vi "Sort-To-XYZ-PRO.vi"(9 "位置 2":i32, 11 "位置":i32) -> (1 "移動二":dbl[](array[numeric]), 3 "移動一":dbl[](array[numeric]), 5 "放球校正?":bool)   [LabVIEW 2019]
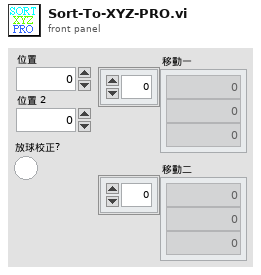
[diagram p1: front panel]
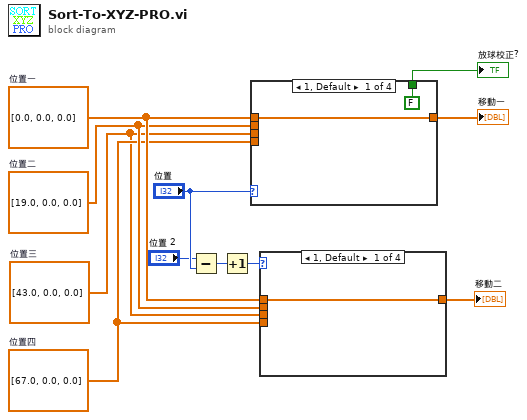
[diagram p0: block diagram]
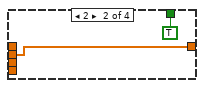
[diagram p5: hidden frame]
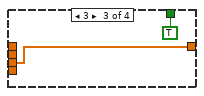
[diagram p6: hidden frame]
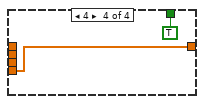
[diagram p7: hidden frame]
diagram:
  w1 = dbl[] [43.0, 0.0, 0.0]  # 位置三
  w8 = dbl[] [67.0, 0.0, 0.0]  # 位置四
  w9 = dbl[] [19.0, 0.0, 0.0]  # 位置二
  w10 = dbl[] [0.0, 0.0, 0.0]  # 位置一
  n1 = Subtract(x="位置 2", y="位置") -> (x-y=w6:i32)
  n2 = Increment(x=w6) -> (x+1=w7:i32)
  n3 = case shown="1, Default" "位置" {
    tunnel: w10 -> [w13 _ _ _]
    tunnel: w9 -> [_ w15 _ _]
    tunnel: w1 -> [_ _ w17 _]
    tunnel: w8 -> [_ _ _ w19]
    tunnel: [w13 w15 w17 w19] -> w11
    tunnel: [FALSE TRUE TRUE TRUE] -> w3
    frame 1, Default {
    }
    frame 2 {
    }
    frame 3 {
    }
    frame 4 {
    }
  }
  "移動一" <- w11
  "放球校正?" <- w3
  n4 = case shown="1, Default" w7 {
    tunnel: w10 -> [w20 _ _ _]
    tunnel: w9 -> [_ w21 _ _]
    tunnel: w1 -> [_ _ w22 _]
    tunnel: w8 -> [_ _ _ w23]
    tunnel: [w20 w21 w22 w23] -> w2
    frame 1, Default {
    }
    frame 2 {
    }
    frame 3 {
    }
    frame 4 {
    }
  }
  "移動二" <- w2
